vi "AlliGator Get Series Analysis Type.vi"(11 "Menu Tag":string) -> (3 "Series Analysis Type":T1)   [LabVIEW 2021, in "AlliGator Scripts.lvlib"]
doc: "Decodes menu tag to determine whether an action is limited to the <B>Current ROI</B> or <B>All ROIs</B>."
uses:
  AlliGator Scripts.lvlib
  AlliGator Series Analysis Type.ctl
panel:
  # "see the AlliGator License on the block diagram (Ctrl+E or Window:Show Block Diagram)"
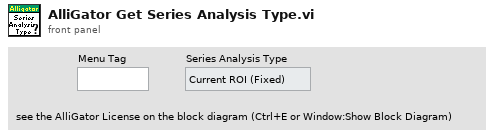
[diagram p1: front panel]
types:
  T1 = typedef "AlliGator Scripts.lvlib/AlliGator Series Analysis Type.ctl" = enum16{"Current ROI (Fixed)", "All ROIs (Fixed)", "Sequential ROIs"}
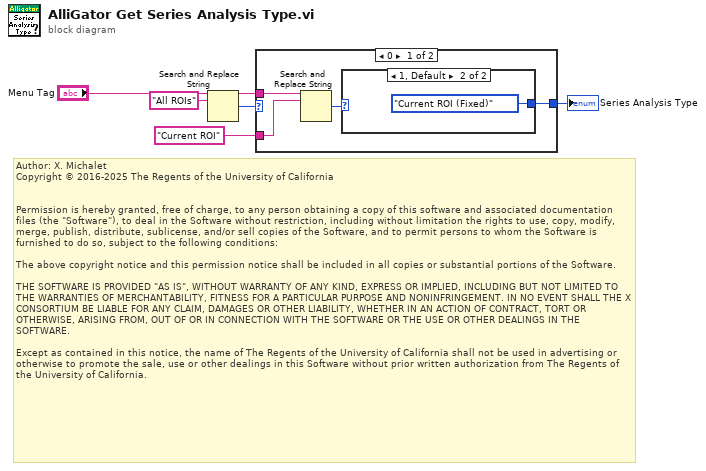
[diagram p0: block diagram]
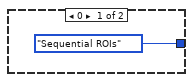
[diagram p2: hidden frame]
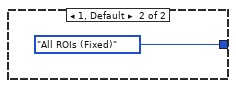
[diagram p3: hidden frame]
diagram:
  # "Author: X. Michalet\nCopyright © 2016-2025 The Regents of the University of California\n \n\nPermission is hereby granted, free of charge, to any person obtaining a copy of this software and associated documentation files (the \"Software\"), to deal in the Software without restriction, including without limitation the rights to use, copy, modify, merge, publish, distribute, sublicense, and/or sell copies of the Software, and to permit persons to whom the Software is furnished to do so, subject to the following conditions:\n\nThe above copyright notice and this permission notice shall be included in all copies or substantial portions of the Software.\n\nTHE SOFTWARE IS PROVIDED \"AS IS\", WITHOUT WARRANTY OF ANY KIND, EXPRESS OR IMPLIED, INCLUDING BUT NOT LIMITED TO THE WARRANTIES OF MERCHANTABILITY, FITNESS FOR A PARTICULAR PURPOSE AND NONINFRINGEMENT. IN NO EVENT SHALL THE X CONSORTIUM BE LIABLE FOR ANY CLAIM, DAMAGES OR OTHER LIABILITY, WHETHER IN AN ACTION OF CONTRACT, TORT OR OTHERWISE, ARISING FROM, OUT OF OR IN CONNECTION WITH THE SOFTWARE OR THE USE OR OTHER DEALINGS IN THE SOFTWARE.\n\nExcept as contained in this notice, the name of The Regents of the University of California shall not be used in advertising or otherwise to promote the sale, use or other dealings in this Software without prior written authorization from The Regents of the University of California."
  n1 = Search and Replace String(input string="Menu Tag", search string="All ROIs") -> (result string=w5:string, number of replacements=w3:i32)  [unwired: 6 in, 2 out]
  n2 = case shown="0" w3 {
    tunnel: [w7 AlliGator_Series_Analysis_Type."All ROIs (Fixed)"] -> w4
    tunnel: w5 -> [w10 _]
    tunnel: "Current ROI" ("search string") -> [w9 _]
    frame 0 {
      n3 = Search and Replace String(input string=w10, search string=w9) -> (number of replacements=w8:i32)  [unwired: 6 in, 3 out]
      n4 = case shown="1, Default" w8 {
        tunnel: [AlliGator_Series_Analysis_Type."Sequential ROIs" AlliGator_Series_Analysis_Type."Current ROI (Fixed)"] -> w7
        frame 0 {
        }
        frame 1, Default {
        }
      }
    }
    frame 1, Default {
    }
  }
  "Series Analysis Type" <- w4
